vi "Chroma2.vi"() -> ()   [LabVIEW 2011]
uses:
  <vilib>/Utility/file.llb/Write To Spreadsheet File (string).vi
panel:
  in  "resource name":refnum<k15>
  out "error out":errorcluster
  in  "seconds to wait":u32
  in  "Name of File":string
  out "Current Data Point":i32
  in  "Interval of Data Collection (sec)":u32
  in  "Type (P_REAL)":i32(ring) items=["P_ENERGY"=4, "P_FACTOR"=3, "P_REACTIVE"=2, "P_APPARENT"=1, "P_REAL"=0]
  in  "Type (I_RMS)":i32(ring) items=["I_THD"=5, "I_CRESTFACTOR"=4, "I_INRUSH"=3, "I_PEAK-"=2, "I_PEAK+"=1, "I_RMS"=0]
  in  "Type (V_RMS)":i32(ring) items=["V_THD"=3, "V_PEAK-"=2, "V_PEAK+"=1, "V_RMS"=0]
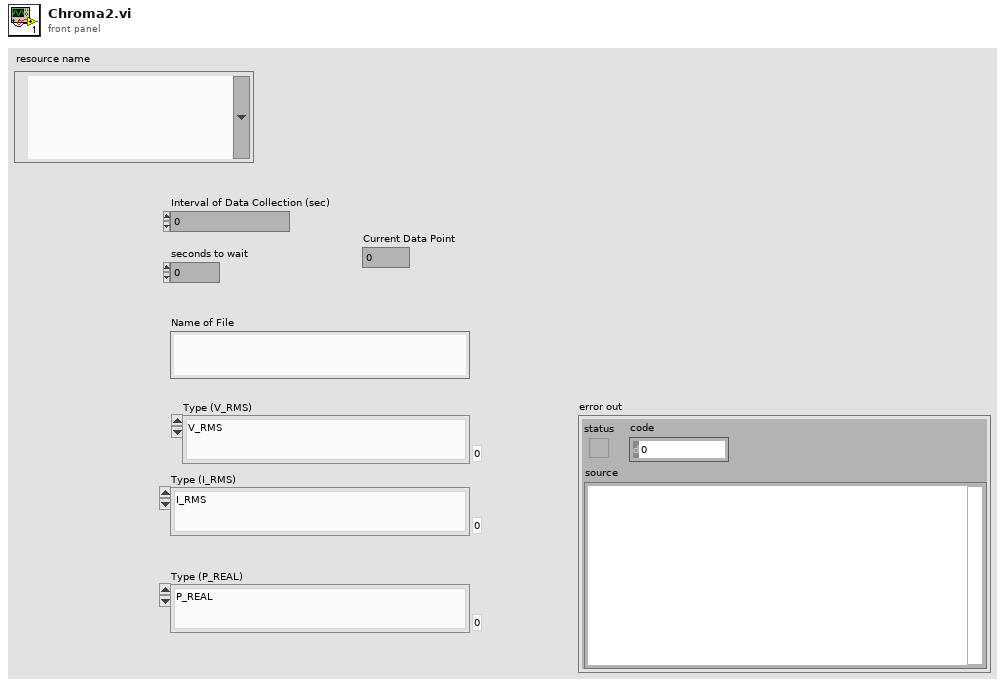
[diagram p1: front panel]
types:
  T1 = enum16{"open", "replace", "create", "open or create", "replace or create", "replace or create with confirmation"}
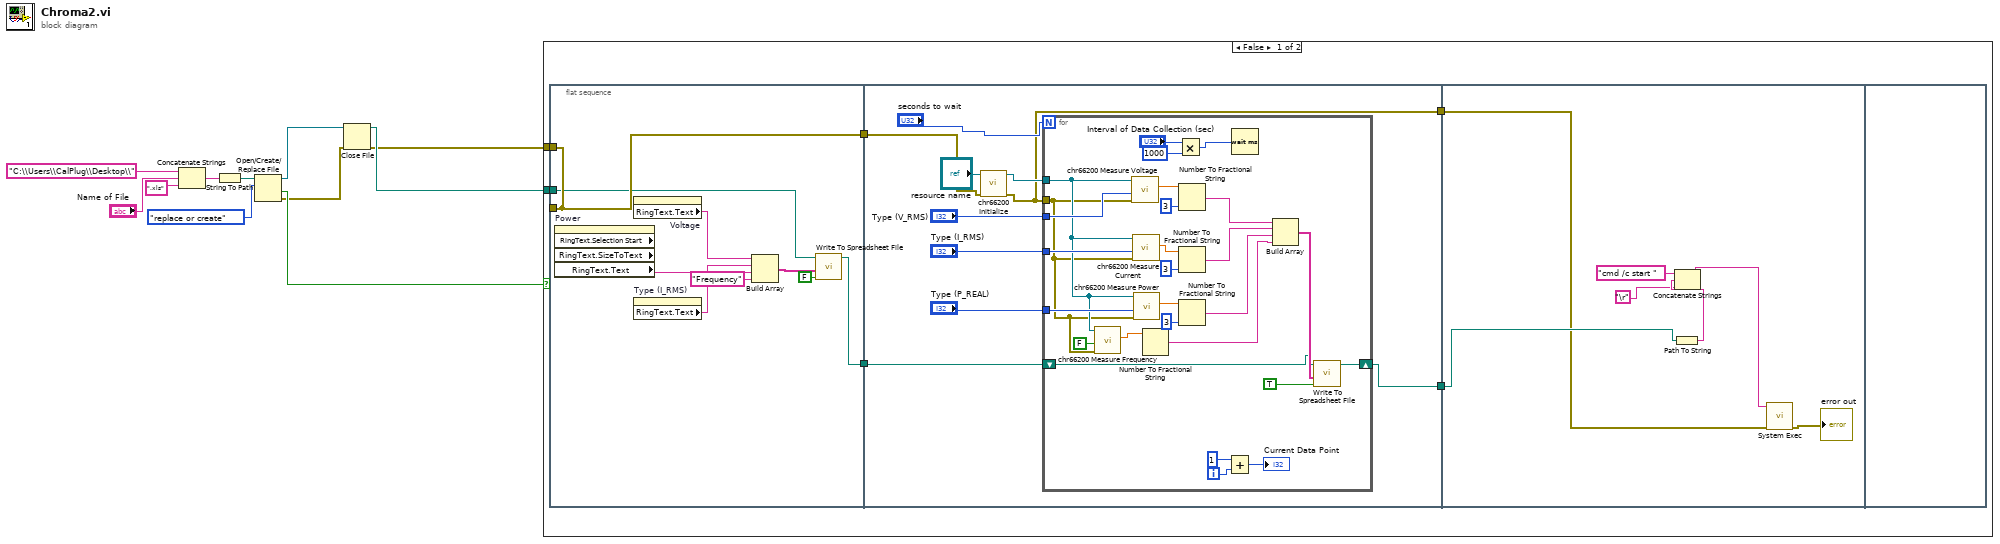
[diagram p0: block diagram]
diagram:
  n1 = Concatenate Strings("C:\\Users\\CalPlug\\Desktop\\" ("string"), "Name of File", ".xls" ("string")) -> (w11:string)
  n2 = String To Path(string=w11) -> (path=w10:path)
  n3 = Open/Create/Replace File(file path (use dialog)=w10, operation (0:open)=T1."replace or create") -> (refnum out=w4:refnum<file>, cancelled=w5:bool, error out=w2:errorcluster)  [unwired: 4 in]
  n4 = Close File(refnum=w4, error in=w2) -> (path=w3:path, error out=w1:errorcluster)
  n5 = case shown="False" w5 {
    tunnel: w3 -> [w15 _]
    tunnel: w1 -> [w12 _]
    frame False {
      n6 = flat-sequence {
        tunnel: [w26] -> w17
        tunnel: [w19] -> w16
        tunnel: [w19] -> _
        tunnel: w15 -> [w18]
        tunnel: w12 -> [w19]
        tunnel: w17 -> [w29]
        tunnel: w16 -> [w32]
        tunnel: [w30] -> w14
        tunnel: [w28] -> w13
        tunnel: w14 -> [w69]
        tunnel: w13 -> [w64]
        frame #0 {
          n7 = property on="Power" class="Ring (strict)" props=["RingText", "Selection Start", "RingText", "SizeToText", "RingText", "Text"]() -> ("RingText.Text"=w23:string)  [unwired: 2 in, 4 out]
          n8 = property on="Voltage" class="Ring (strict)"() -> ("RingText.Text"=w24:string)  [unwired: 2 in, 2 out]
          n9 = property on="Type (I_RMS)" class="Ring (strict)"() -> ("RingText.Text"=w22:string)  [unwired: 2 in, 2 out]
          n10 = Build Array(w24, w22, w23, "Frequency" ("element")) -> (w21:string[])
          n11 = call-poly <vilib>:"Write To Spreadsheet File.vi"("append to file? (new file:F)"=FALSE, "1D data"=w21, "file path (dialog if empty)"=w18) -> ("new file path (Not A Path if cancelled)"=w26:path)  [unwired: 5 in]
        }
        frame #1 {
          n12 = call <instrlib>:"chr66200 Initialize.vi"("error in (no error)"=w32, "resource name"="resource name") -> ("error out"=w28:errorcluster, "instrument handle out"=w33:refnum<k15>)  [unwired: 8 in]
          n13 = for {
            N: "seconds to wait" -> [_]
            tunnel: w33 -> [w43]
            tunnel: w28 -> [w38]
            tunnel: "Type (I_RMS)" -> [w63]
            tunnel: "Type (V_RMS)" -> [w62]
            tunnel: "Type (P_REAL)" -> [w61]
            shift-right: [w60] -> w30
            shift-left: w29 -> [w37]
            i -> [w51]
            n14 = call <instrlib>:"chr66200 Measure Frequency.vi"("error in (no error)"=w38, "Measure Fetch (Fetch)"=FALSE, "instrument handle"=w43) -> ("Read Value"=w41:dbl)  [unwired: 6 in, 2 out]
            n15 = call <instrlib>:"chr66200 Measure Voltage.vi"("error in (no error)"=w38, "Type (V_RMS)"=w62, "instrument handle"=w43) -> ("Read Value"=w58:dbl)  [unwired: 6 in, 2 out]
            n16 = call <instrlib>:"chr66200 Measure Current.vi"("error in (no error)"=w38, "Type (I_RMS)"=w63, "instrument handle"=w43) -> ("Read Value"=w57:dbl)  [unwired: 6 in, 2 out]
            n17 = call <instrlib>:"chr66200 Measure Power.vi"("error in (no error)"=w38, "Type (P_REAL)"=w61, "instrument handle"=w43) -> ("Read Value"=w56:dbl)  [unwired: 6 in, 2 out]
            n18 = Number To Fractional String(number=w41) -> (F-format string=w39:string)  [unwired: 3 in]
            n19 = Multiply(x="Interval of Data Collection (sec)", y=u32 1000) -> (x*y=w46:u32)
            n20 = Number To Fractional String(number=w58, precision (6)=i16 3) -> (F-format string=w45:string)  [unwired: 2 in]
            n21 = Number To Fractional String(number=w57, precision (6)=i16 3) -> (F-format string=w44:string)  [unwired: 2 in]
            n22 = Number To Fractional String(number=w56, precision (6)=i16 3) -> (F-format string=w40:string)  [unwired: 2 in]
            n23 = Add(x=1, y=w51) -> (x+y=→"Current Data Point":i32)
            n24 = Wait (ms)(milliseconds to wait=w46) -> ()  [unwired: 1 out]
            n25 = Build Array(w45, w44, w40, w39) -> (w52:string[])
            n26 = call-poly <vilib>:"Write To Spreadsheet File.vi"("append to file? (new file:F)"=TRUE, "1D data"=w52, "file path (dialog if empty)"=w37) -> ("new file path (Not A Path if cancelled)"=w60:path)  [unwired: 5 in]
          }
        }
        frame #2 {
          n27 = Path To String(path=w69) -> (string=w68:string)
          n28 = Concatenate Strings("cmd /c start " ("string"), w68, "\r") -> (w66:string)
          n29 = call <vilib>:"System Exec.vi"("error in (no error)"=w64, "command line"=w66) -> ("error out"=→"error out":errorcluster)  [unwired: 6 in, 3 out]
        }
        frame #3 {
        }
      }
    }
    frame True {
    }
  }
